vi "Execute.vi"(8 "error in (no error)":errorcluster, 10 "Plugin Handler Stop in":refnum<class "Plugin Handler Stop.lvclass">, 11 "Plugin Handler Shifter Data Definition":T1) -> (0 "error out":errorcluster, 1 "Stop?":bool, 2 "Plugin Generic Command out":refnum<class "Plugin Handler Command.lvclass">, 3 "Plugin Handler Shifter Data Out":T1)   [LabVIEW 2011, in "Plugin Handler Stop.lvclass"]
uses:
  Plugin Handler Stop.lvclass
  Plugin Handler Command.lvclass
  Plugin Strict Type Definitions/Plugin Handler Shifter Data Definition.ctl
  Parent Plugin Definition/Plugin Template/Generic Plugin.lvclass
  Plugin Strict Type Definitions/Plugin Configuration Information.ctl
  User Interface/UI Command Manager/UI Command Manager.lvclass
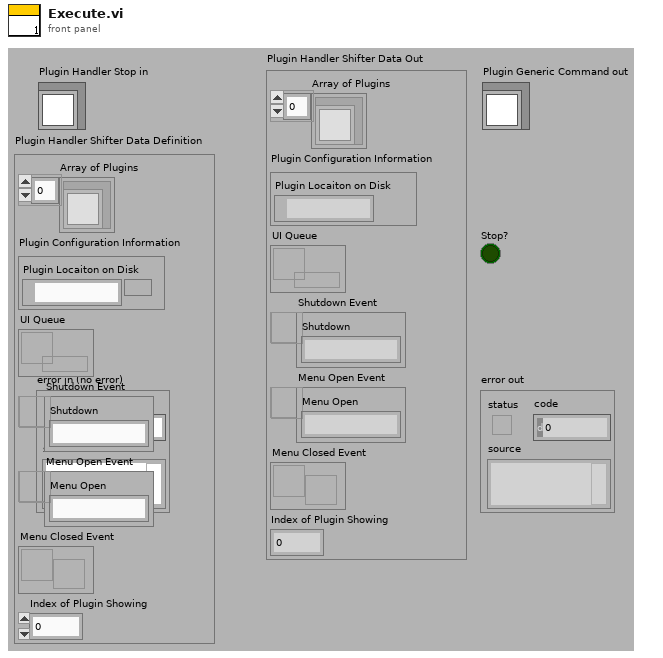
[diagram p1: front panel]
types:
  T1 = typedef "Plugin Handler Shifter Data Definition.ctl" = cluster{"Array of Plugins":refnum<class "Generic Plugin.lvclass">[], "Plugin Configuration Information":T2, "UI Queue":refnum<queue>, "Shutdown Event":refnum<user-event>, "Menu Open Event":refnum<user-event>, "Menu Closed Event":refnum<user-event>, "Index of Plugin Showing":i32}
  T2 = typedef "Plugin Configuration Information.ctl" = cluster{"Plugin Locaiton on Disk":path}
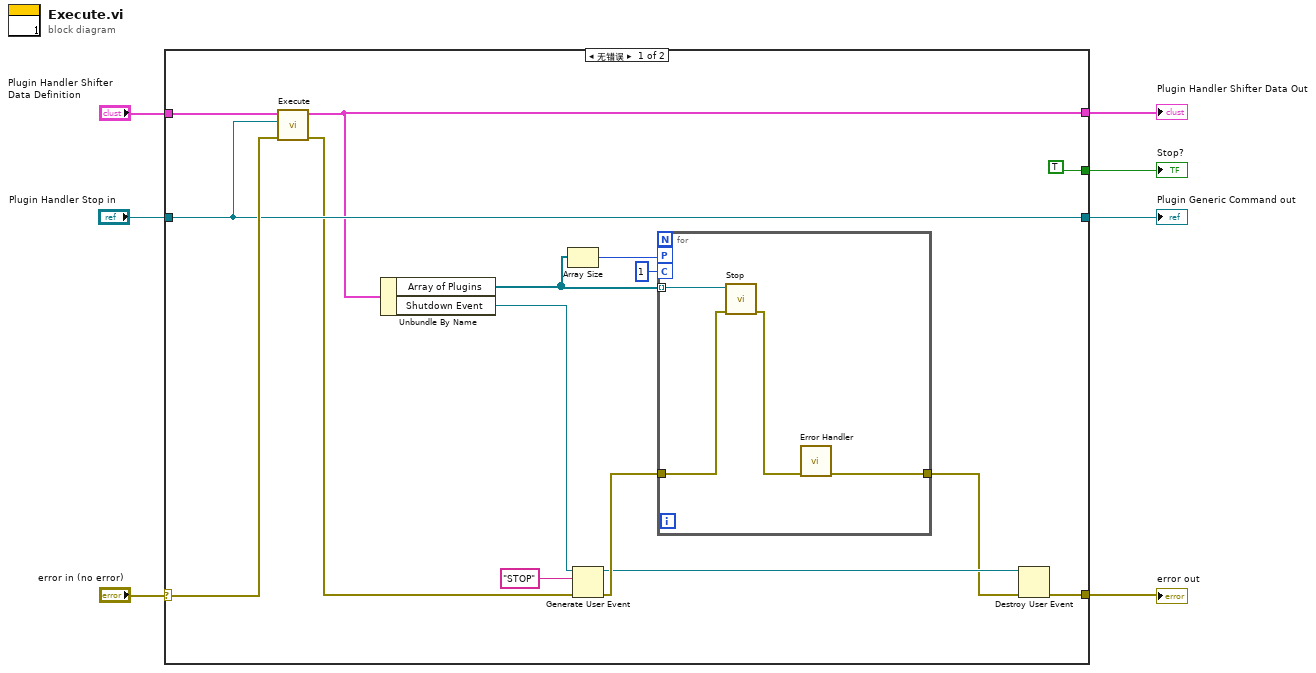
[diagram p0: block diagram]
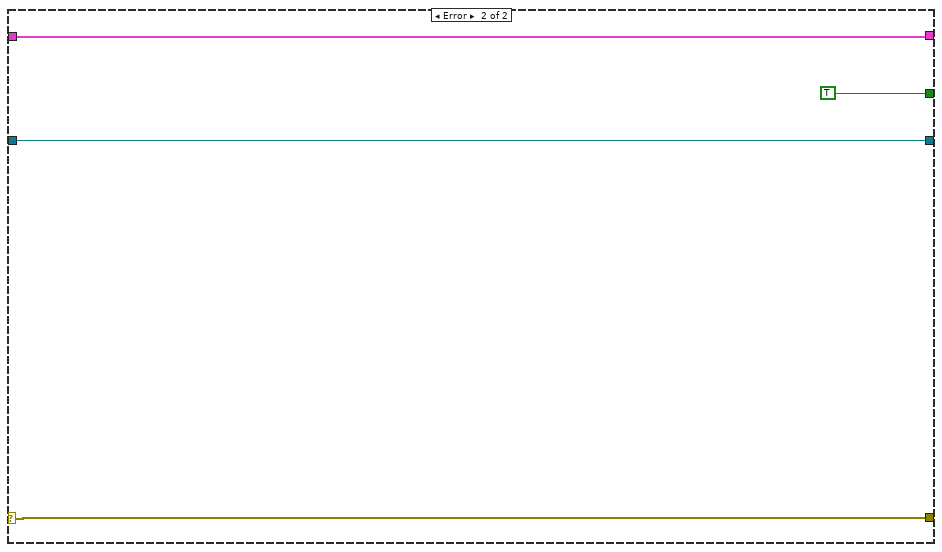
[diagram p2: hidden frame]
diagram:
  n1 = case shown="无错误" "error in (no error)" {
    selector: "error in (no error)" -> [w22 w29]
    tunnel: "Plugin Handler Stop in" -> [w20 w30]
    tunnel: "Plugin Handler Shifter Data Definition" -> [w21 w28]
    tunnel: [w20 w30] -> w4
    tunnel: [w9 w29] -> w3
    tunnel: [w16 w28] -> w2
    tunnel: [TRUE TRUE] -> w1
    frame No Error {
      n2 = call-parent "Execute.vi"("error in (no error)"=w22, "Plugin Generic Command in"=w20, "Plugin Handler Shifter Data Definition"=w21) -> ("error out"=w17:errorcluster, "Plugin Handler Shifter Data Out"=w16:T1)  [unwired: 5 in, 2 out]
      n3 = Unbundle By Name(w16) -> ("Array of Plugins"=w15:refnum<class "Generic Plugin.lvclass">[], "Shutdown Event"=w18:refnum<user-event>)
      n4 = Array Size(array=w15) -> (size(s)=w14:i32)
      n5 = Generate User Event(user event=w18, event data cluster="STOP" ("event data"), error in=w17) -> (user event out=w11:refnum<user-event>, error out=w12:errorcluster)
      n6 = for {
        tunnel: w15 -> [w26] mode=indexing
        workers-P: w14 -> [_]
        chunk-C: 1 -> [_]
        tunnel: w12 -> [w25]
        tunnel: [w23] -> w10
        n7 = call-dynamic "Stop.vi"("error out"=w25, "Generic Plugin in"=w26) -> ("error IO"=w24:errorcluster)  [unwired: 7 in, 2 out]
        n8 = call "Error Handler.vi"("error in (no error)"=w24) -> ("error out"=w23:errorcluster)  [unwired: 10 in]
      }
      n9 = Destroy User Event(user event=w11, error in=w10) -> (error out=w9:errorcluster)
    }
    frame Error {
    }
  }
  "Plugin Generic Command out" <- w4
  "Stop?" <- w1
  "Plugin Handler Shifter Data Out" <- w2
  "error out" <- w3
